vi "Acquire.vi"(8 "error in (no error)":errorcluster, 9 "Initialize":bool, 10 "Reply to":refnum<class "Result Reply Msg.lvclass">, 11 "Measure Controller in":refnum<class "Measure Controller.lvclass">) -> (0 "error out":errorcluster, 3 "Measure Controller out":refnum<class "Measure Controller.lvclass">)   [LabVIEW 2015, in "Measure Controller.lvclass"]
uses:
  Measure Controller.lvclass
  Measure Object Messages/Result Reply Msg/Result Reply Msg.lvclass
  Measure Controller Messages/Result Response Msg/Result Response Msg.lvclass
  Measure Object/Measure Object.lvclass/Measure Object.ctl
  Results/Acquired Result/Acquired Result.lvclass
  Measure Object Messages/Write tdms stream Msg/Write tdms stream Msg.lvclass/Write tdms stream Msg.ctl
  <vilib>/ActorFramework/Message Enqueuer/Message Enqueuer.lvclass/Message Enqueuer.ctl
  Measure Object Messages/Acquire Msg/Acquire Msg.lvclass/Acquire Msg.ctl
  Measure Controller.lvclass/Measure Controller.ctl
  Measure Object/Read tdms stream.vi
  <vilib>/ActorFramework/Message Enqueuer/Enqueue.vi
  <vilib>/ActorFramework/Message Priority Queue/Priority Enqueue.vi
  Measure Object Messages/Write tdms stream Msg/Write tdms stream Msg.lvclass
  Measure Object Messages/Acquire Msg/Acquire Msg.lvclass
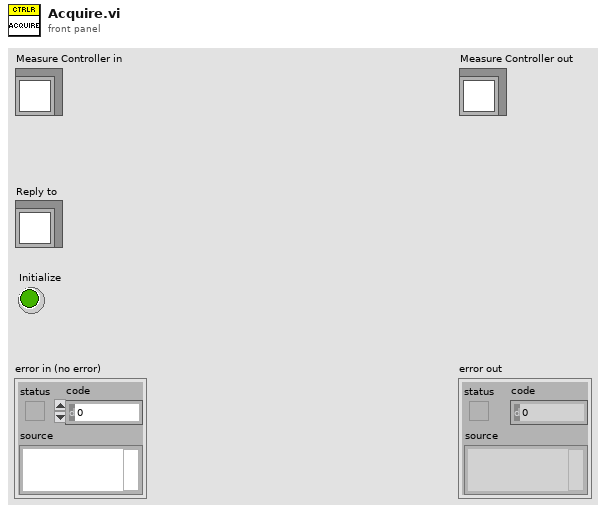
[diagram p1: front panel]
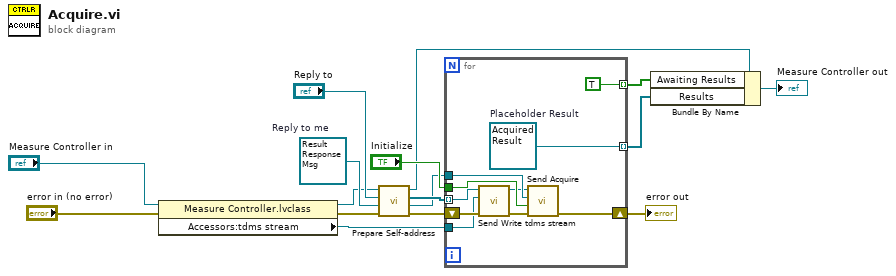
[diagram p0: block diagram]
diagram:
  w6 = refnum<class "Result Response Msg.lvclass"> refnum  # Reply to me
  n1 = property class="Measure Controller.lvclass"(reference="Measure Controller in", error in="error in (no error)") -> (reference out=w5:refnum<class "Measure Controller.lvclass">, error out=w2:errorcluster, "Accessors:tdms stream"=w4:refnum<k34>)
  n2 = call-dynamic "Prepare Self-address.vi"("error in (no error)"=w2, "Reply to me"=w6, "Reply to"="Reply to", "Measure Controller in"=w5) -> ("error out"=w1:errorcluster, "Reply to me"=w7:refnum<class "Result Reply Msg.lvclass">, "Active measurements enqueuers"=w8:refnum<class "Message Enqueuer.lvclass">[], "Measure Controller out"=w9:refnum<class "Measure Controller.lvclass">)  [unwired: 4 in]
  n3 = for {
    shift-right: [w26] -> w13
    shift-left: w1 -> [w19]
    tunnel: "Initialize" -> [w23]
    tunnel: [TRUE] -> w16 mode=indexing
    tunnel: [w24] -> w15 mode=indexing
    tunnel: w8 -> [w21] mode=indexing
    tunnel: w7 -> [w22]
    tunnel: w4 -> [w17]
    w24 = refnum<class "Acquired Result.lvclass"> refnum  # Placeholder Result
    n4 = call "Send Write tdms stream.vi"("error in (no error)"=w19, "tdms stream"=w17, "Message Enqueuer"=w21) -> ("error out"=w18:errorcluster, "Message Enqueuer out"=w20:refnum<class "Message Enqueuer.lvclass">)  [unwired: 7 in]
    n5 = call "Send Acquire.vi"("error in (no error)"=w18, "Initialize"=w23, "Reply to"=w22, "Message Enqueuer"=w20) -> ("error out"=w26:errorcluster)  [unwired: 6 in, 1 out]
  }
  "error out" <- w13
  n6 = Bundle By Name(cluster=w9, "Awaiting Results"=w16, "Results"=w15) -> (→"Measure Controller out":refnum<class "Measure Controller.lvclass">)
